vi "3_Cell_Test.vi"() -> ()   [LabVIEW 2020]
uses:
  Drivers-Essentials/global stop1.vi
  Drivers-Essentials/Global Stop 2.vi
  Global_Stop_3.vi
panel:
  out "Battery 3 Current":dbl(graph)
  out "Battery 1 Current":dbl(graph)
  out "Battery 3 Temperature":dbl(graph)
  out "Battery 3 Strain":dbl(graph)
  out "Battery 3 Voltage":dbl(graph)
  out "Battery 2 Temperature":dbl(graph)
  out "Battery 2 Strain":dbl(graph)
  out "Battery 1 Temperature":dbl(graph)
  out "Battery 1 Strain":dbl(graph)
  out "Battery 2 Voltage":dbl(graph)
  out "Battery 1 Voltage":dbl(graph)
  out "Battery 2 Current":dbl(graph)
  out "PS VIS resource name out 3":refnum<visa-resource-name>
  out "PS error out 3":errorcluster
  in  "NHR error in 3":errorcluster
  out "PS VIS resource name out 2":refnum<visa-resource-name>
  out "PS error out 2":errorcluster
  in  "NHR error in 2":errorcluster
  out "PS error out":errorcluster
  out "PS VIS resource name out":refnum<visa-resource-name>
  in  "NHR error in":errorcluster
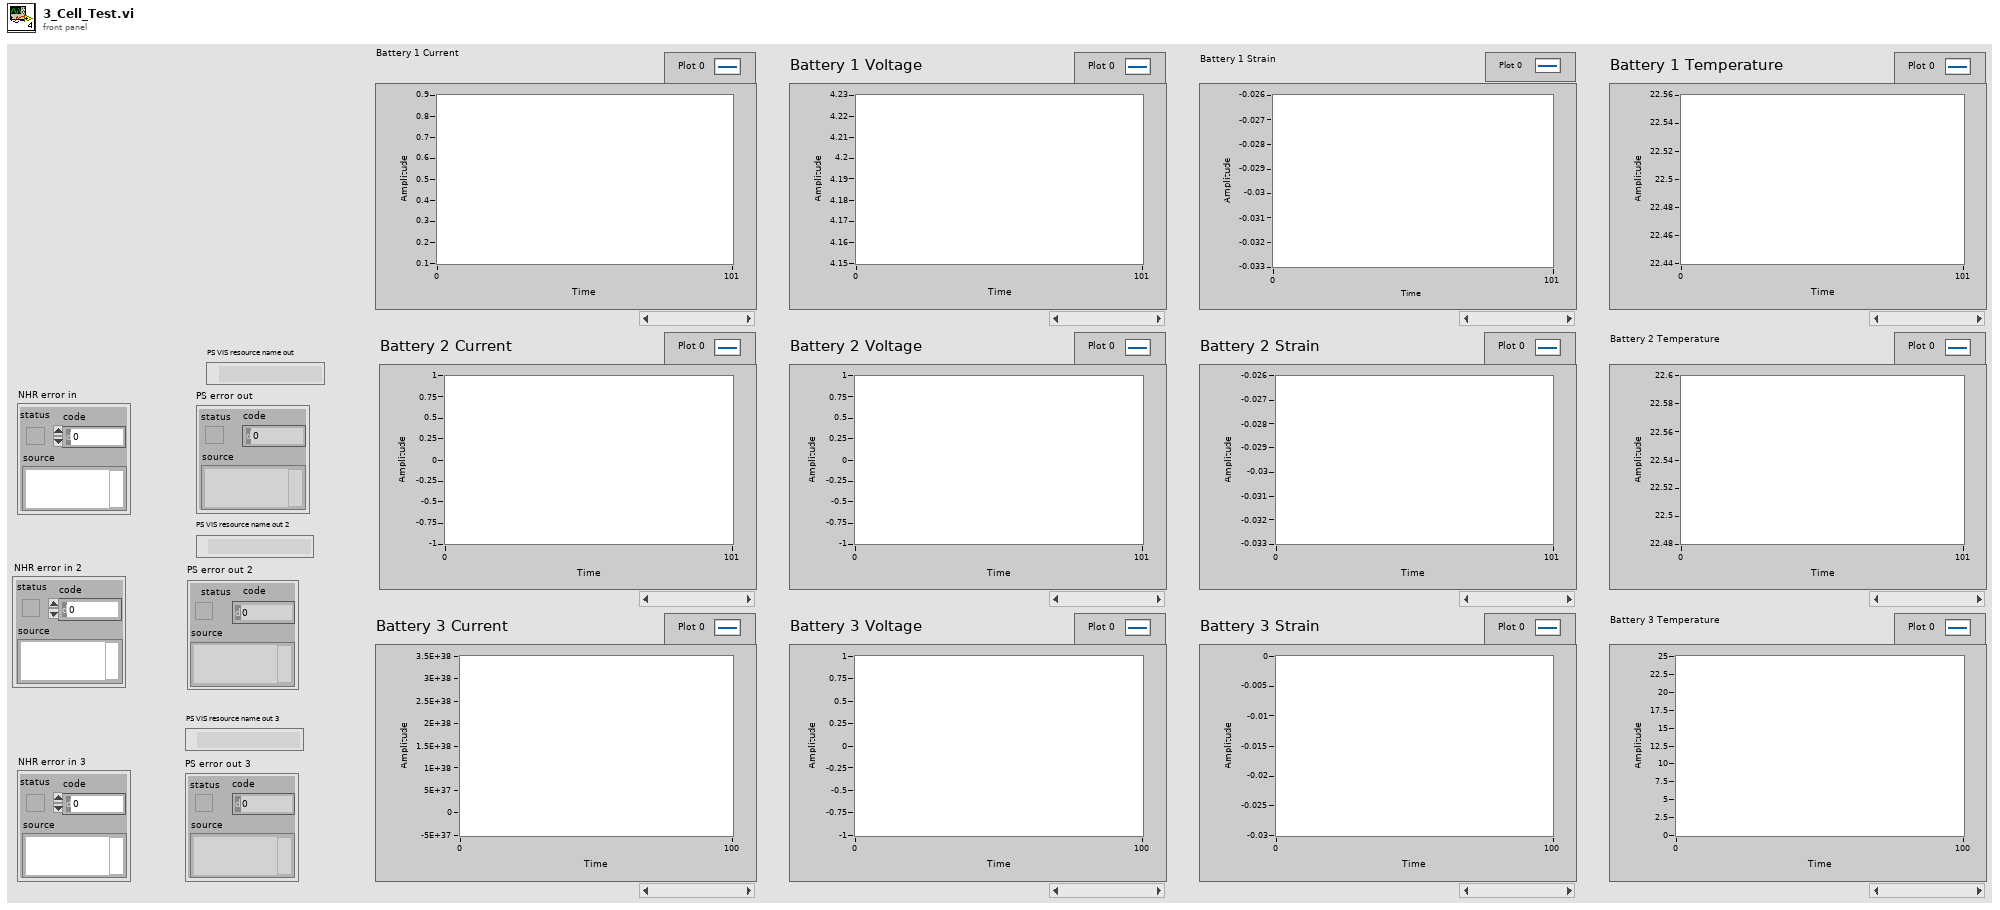
[diagram p1: front panel]
types:
  T1 = cluster{"Min Voltage (V)":dbl, "Min Voltage Time (s)":dbl, "Max Voltage (V)":dbl, "Max Voltage Time (s)":dbl, "Max Sink Current (A)":dbl, "Max Sink Current Time (s)":dbl, "Max Source Current (A)":dbl, "Max Source Current Time (s)":dbl, "Max Sink Power (W)":dbl, "Max Sink Power Time (s)":dbl, "Max Source Power (W)":dbl, "Max Source Power Time (s)":dbl}
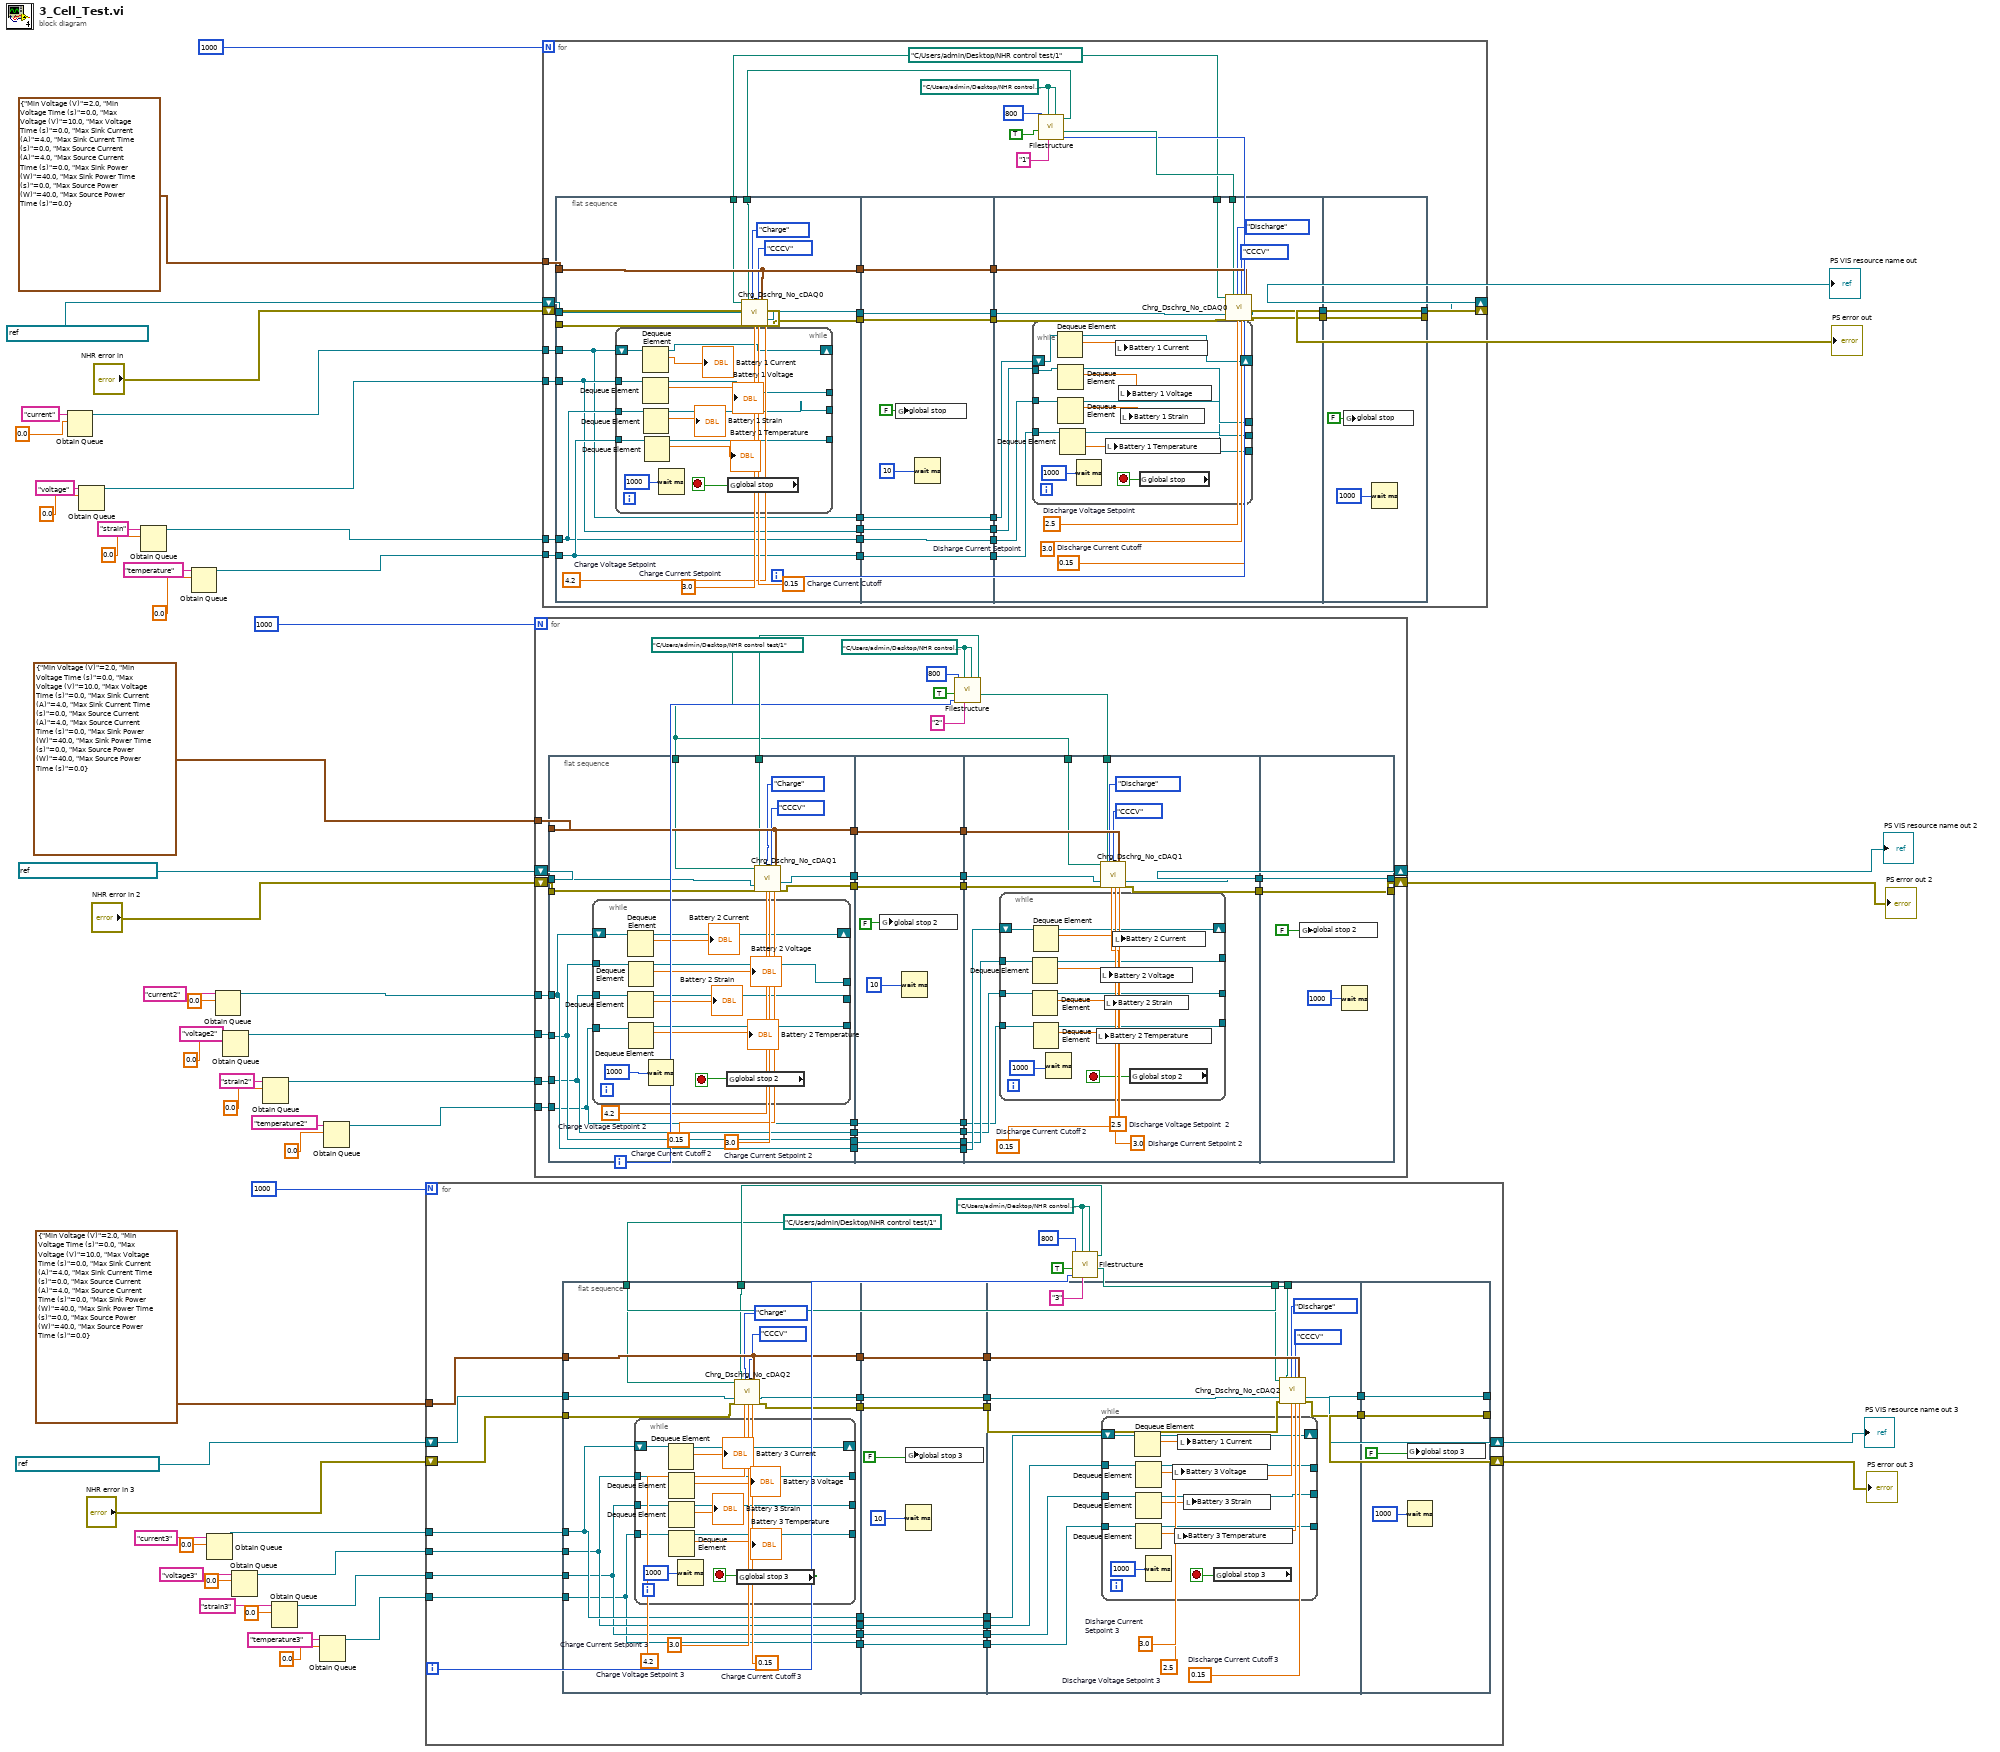
[diagram p0: block diagram]
diagram:
  n1 = Obtain Queue(name (unnamed)="current", element data type=0.0) -> (queue out=w34:refnum<queue>)  [unwired: 3 in, 2 out]
  n2 = Obtain Queue(name (unnamed)="voltage", element data type=0.0) -> (queue out=w25:refnum<queue>)  [unwired: 3 in, 2 out]
  n3 = Obtain Queue(name (unnamed)="strain", element data type=0.0) -> (queue out=w19:refnum<queue>)  [unwired: 3 in, 2 out]
  n4 = Obtain Queue(name (unnamed)="temperature", element data type=0.0) -> (queue out=w16:refnum<queue>)  [unwired: 3 in, 2 out]
  n5 = Obtain Queue(name (unnamed)="current3", element data type=0.0) -> (queue out=w28:refnum<queue>)  [unwired: 3 in, 2 out]
  n6 = Obtain Queue(name (unnamed)="current2", element data type=0.0) -> (queue out=w31:refnum<queue>)  [unwired: 3 in, 2 out]
  n7 = Obtain Queue(name (unnamed)="voltage2", element data type=0.0) -> (queue out=w22:refnum<queue>)  [unwired: 3 in, 2 out]
  n8 = Obtain Queue(name (unnamed)="voltage3", element data type=0.0) -> (queue out=w7:refnum<queue>)  [unwired: 3 in, 2 out]
  n9 = Obtain Queue(name (unnamed)="strain2", element data type=0.0) -> (queue out=w13:refnum<queue>)  [unwired: 3 in, 2 out]
  n10 = Obtain Queue(name (unnamed)="strain3", element data type=0.0) -> (queue out=w4:refnum<queue>)  [unwired: 3 in, 2 out]
  n11 = Obtain Queue(name (unnamed)="temperature3", element data type=0.0) -> (queue out=w1:refnum<queue>)  [unwired: 3 in, 2 out]
  n12 = Obtain Queue(name (unnamed)="temperature2", element data type=0.0) -> (queue out=w10:refnum<queue>)  [unwired: 3 in, 2 out]
  n13 = for {
    N: 1000 -> [_]
    tunnel: T1 {"Min Voltage (V)"=2.0, "Min Voltage Time (s)"=0.0, "Max Voltage (V)"=10.0, "Max Voltage Time (s)"=0.0, "Max Sink Current (A)"=4.0, "Max Sink Current Time (s)"=0.0, "Max Source Current (A)"=4.0, "Max Source Current Time (s)"=0.0, "Max Sink Power (W)"=40.0, "Max Sink Power Time (s)"=0.0, "Max Source Power (W)"=40.0, "Max Source Power Time (s)"=0.0} ("Output Safety") -> [w79]
    shift-right: [w85] -> w44
    shift-left: "NHR error in 3" -> [w87]
    shift-right: [w84] -> w43
    shift-left: refnum<visa-resource-name> "TCPIP0::192.168.0.94::inst0::INSTR" ("NHR VISA 3") -> [w86]
    tunnel: w28 -> [w64]
    tunnel: w7 -> [w63]
    tunnel: w4 -> [w60]
    tunnel: w1 -> [w57]
    i -> [w76]
    w75 = path "C:/Users/admin/Desktop/NHR control test/1" ("file path (use dialog)")
    w80 = path "C:/Users/admin/Desktop/NHR control test" ("filepath 3")
    n14 = flat-sequence {
      tunnel: [w103] -> w74
      tunnel: [w102] -> w72
      tunnel: [w101] -> w70
      tunnel: w79 -> [w103]
      tunnel: w87 -> [w95]
      tunnel: w86 -> [w94]
      tunnel: w78 -> [w93]
      tunnel: w75 -> [w92]
      tunnel: w64 -> [w91]
      tunnel: [w91] -> w68
      tunnel: w63 -> [w90]
      tunnel: [w90] -> w61
      tunnel: w60 -> [w89]
      tunnel: [w89] -> w58
      tunnel: w57 -> [w88]
      tunnel: [w88] -> w55
      tunnel: w74 -> [w126]
      tunnel: [w126] -> w73
      tunnel: w72 -> [w125]
      tunnel: [w125] -> w71
      tunnel: w70 -> [w124]
      tunnel: [w124] -> w69
      tunnel: w68 -> [w123]
      tunnel: [w123] -> w67
      tunnel: [w120] -> w62
      tunnel: w61 -> [w120]
      tunnel: [w119] -> w59
      tunnel: w58 -> [w119]
      tunnel: [w118] -> w56
      tunnel: w55 -> [w118]
      tunnel: w73 -> [w137]
      tunnel: w71 -> [w134]
      tunnel: w69 -> [w133]
      tunnel: w77 -> [w132]
      tunnel: w75 -> [w131]
      tunnel: w67 -> [w129]
      tunnel: [w139] -> w66
      tunnel: [w138] -> w65
      tunnel: w62 -> [w130]
      tunnel: w59 -> [w127]
      tunnel: w56 -> [w128]
      tunnel: [w159] -> w84
      tunnel: [w160] -> w85
      tunnel: w66 -> [w160]
      tunnel: w65 -> [w159]
      frame #0 {
        w100 = 0.15  # Charge Current Cutoff 3
        w99 = 3.0  # Charge Current Setpoint 3
        w98 = 4.2  # Charge Voltage Setpoint 3
        n15 = while {
          tunnel: [w115] -> _
          tunnel: [w114] -> _
          tunnel: [w113] -> _
          shift-right: [w108] -> _
          shift-left: w91 -> [w109]
          tunnel: w90 -> [w107]
          tunnel: w88 -> [w106]
          tunnel: w89 -> [w105]
          stop <- w116 stop-if-true
          n16 = Dequeue Element(queue=w109) -> (queue out=w108:refnum<queue>, element=→"Battery 3 Current":dbl)  [unwired: 2 in, 2 out]
          n17 = Dequeue Element(queue=w107) -> (queue out=w115:refnum<queue>, element=→"Battery 3 Voltage":dbl)  [unwired: 2 in, 2 out]
          n18 = Dequeue Element(queue=w105) -> (queue out=w114:refnum<queue>, element=→"Battery 3 Strain":dbl)  [unwired: 2 in, 2 out]
          n19 = Dequeue Element(queue=w106) -> (queue out=w113:refnum<queue>, element=→"Battery 3 Temperature":dbl)  [unwired: 2 in, 2 out]
          n20 = Wait (ms)(milliseconds to wait=1000) -> ()  [unwired: 1 out]
          n21 = global read "Global_Stop_3.vi" "global stop 3"() -> (w116:bool)
        }
        n22 = call "Chrg_Dschrg_No_cDAQ2.vi"("file path (use dialog)"=w92, "PS VISA in"=w94, "PS error in"=w95, "DischargeCyclePath"=w93, "Charge/discharge"=enum8{"Charge", "Discharge"}."Charge", "Charge/Discharge Voltage Setpoint"=w98, "CC or CCCV"=enum16{"CC", "CCCV"}."CCCV", "Current Setpoint"=w99, "Output Safety"=w103, "Current Cutoff"=w100) -> ("PS VIS resource name out"=w102:refnum<visa-resource-name>, "PS error out"=w101:errorcluster)  [unwired: 8 in]
      }
      frame #1 {
        n23 = global write "Global_Stop_3.vi" "global stop 3"(FALSE ("global stop")) -> ()
        n24 = Wait (ms)(milliseconds to wait=10) -> ()  [unwired: 1 out]
      }
      frame #2 {
        w141 = 3.0  # Disharge Current Setpoint 3
        w142 = 0.15  # Discharge Current Cutoff 3
        w140 = 2.5  # Discharge Voltage Setpoint 3
        n25 = while {
          tunnel: [w154] -> _
          tunnel: [w152] -> _
          tunnel: [w150] -> _
          shift-right: [w147] -> _
          shift-left: w129 -> [w148]
          tunnel: w130 -> [w146]
          tunnel: w128 -> [w145]
          tunnel: w127 -> [w144]
          stop <- w155 stop-if-true
          n26 = Dequeue Element(queue=w148) -> (queue out=w147:refnum<queue>, element=w143:dbl)  [unwired: 2 in, 2 out]
          n27 = Dequeue Element(queue=w146) -> (queue out=w154:refnum<queue>, element=w153:dbl)  [unwired: 2 in, 2 out]
          n28 = Dequeue Element(queue=w144) -> (queue out=w152:refnum<queue>, element=w151:dbl)  [unwired: 2 in, 2 out]
          n29 = Dequeue Element(queue=w145) -> (queue out=w150:refnum<queue>, element=w149:dbl)  [unwired: 2 in, 2 out]
          n30 = Wait (ms)(milliseconds to wait=1000) -> ()  [unwired: 1 out]
          n31 = local write "Battery 3 Voltage"(w153) -> ()
          n32 = local write "Battery 3 Temperature"(w149) -> ()
          n33 = local write "Battery 1 Current"(w143) -> ()
          n34 = local write "Battery 3 Strain"(w151) -> ()
          n35 = global read "Global_Stop_3.vi" "global stop 3"() -> (w155:bool)
        }
        n36 = call "Chrg_Dschrg_No_cDAQ2.vi"("file path (use dialog)"=w131, "PS VISA in"=w134, "PS error in"=w133, "DischargeCyclePath"=w132, "Charge/discharge"=enum8{"Charge", "Discharge"}."Discharge", "Charge/Discharge Voltage Setpoint"=w140, "CC or CCCV"=enum16{"CC", "CCCV"}."CCCV", "Current Setpoint"=w141, "Output Safety"=w137, "Current Cutoff"=w142) -> ("PS VIS resource name out"=w138:refnum<visa-resource-name>, "PS error out"=w139:errorcluster)  [unwired: 8 in]
      }
      frame #3 {
        n37 = global write "Global_Stop_3.vi" "global stop 3"(FALSE ("global stop")) -> ()
        n38 = Wait (ms)(milliseconds to wait=1000) -> ()  [unwired: 1 out]
      }
    }
    n39 = call "Filestructure.vi"("Discharge filepath"=w80, "Batteryname"="3" ("Batteryname 3"), "Charge filepath"=w80, "For loop i"=w76, "In for loop"=TRUE, "Starting Cycle"=800 ("Starting Cycle 3")) -> ("DischargeCyclePath"=w77:path, "ChargeCyclePath"=w78:path)  [unwired: 1 in, 3 out]
  }
  "PS error out 3" <- w44
  "PS VIS resource name out 3" <- w43
  n40 = for {
    N: 1000 -> [_]
    tunnel: T1 {"Min Voltage (V)"=2.0, "Min Voltage Time (s)"=0.0, "Max Voltage (V)"=10.0, "Max Voltage Time (s)"=0.0, "Max Sink Current (A)"=4.0, "Max Sink Current Time (s)"=0.0, "Max Source Current (A)"=4.0, "Max Source Current Time (s)"=0.0, "Max Sink Power (W)"=40.0, "Max Sink Power Time (s)"=0.0, "Max Source Power (W)"=40.0, "Max Source Power Time (s)"=0.0} ("Output Safety") -> [w185]
    shift-right: [w191] -> w48
    shift-left: "NHR error in 2" -> [w193]
    shift-right: [w190] -> w47
    shift-left: refnum<visa-resource-name> "TCPIP0::192.168.0.93::inst0::INSTR" ("NHR VISA 2") -> [w192]
    tunnel: w31 -> [w163]
    tunnel: w22 -> [w172]
    tunnel: w13 -> [w171]
    tunnel: w10 -> [w166]
    i -> [w182]
    w181 = path "C:/Users/admin/Desktop/NHR control test/1" ("file path (use dialog)")
    w186 = path "C:/Users/admin/Desktop/NHR control test" ("filepath 2")
    n41 = flat-sequence {
      tunnel: [w207] -> w180
      tunnel: [w209] -> w178
      tunnel: [w208] -> w176
      tunnel: w185 -> [w209]
      tunnel: w193 -> [w202]
      tunnel: w192 -> [w203]
      tunnel: w183 -> [w199]
      tunnel: w181 -> [w198]
      tunnel: w172 -> [w196]
      tunnel: w171 -> [w195]
      tunnel: [w196] -> w169
      tunnel: [w195] -> w167
      tunnel: w166 -> [w194]
      tunnel: [w194] -> w164
      tunnel: w163 -> [w197]
      tunnel: [w197] -> w161
      tunnel: w180 -> [w232]
      tunnel: [w232] -> w179
      tunnel: w178 -> [w231]
      tunnel: [w231] -> w177
      tunnel: w176 -> [w230]
      tunnel: [w230] -> w175
      tunnel: [w227] -> w170
      tunnel: w169 -> [w227]
      tunnel: [w226] -> w168
      tunnel: w167 -> [w226]
      tunnel: [w225] -> w165
      tunnel: w164 -> [w225]
      tunnel: [w224] -> w162
      tunnel: w161 -> [w224]
      tunnel: w179 -> [w243]
      tunnel: w177 -> [w241]
      tunnel: w184 -> [w238]
      tunnel: w175 -> [w242]
      tunnel: w181 -> [w237]
      tunnel: [w245] -> w174
      tunnel: [w244] -> w173
      tunnel: w170 -> [w235]
      tunnel: w168 -> [w234]
      tunnel: w165 -> [w233]
      tunnel: w162 -> [w236]
      tunnel: [w265] -> w190
      tunnel: [w266] -> w191
      tunnel: w174 -> [w266]
      tunnel: w173 -> [w265]
      frame #0 {
        w204 = 0.15  # Charge Current Cutoff 2
        w205 = 3.0  # Charge Current Setpoint 2
        w206 = 4.2  # Charge Voltage Setpoint 2
        n42 = while {
          tunnel: [w220] -> _
          tunnel: [w218] -> _
          tunnel: [w216] -> _
          shift-right: [w213] -> _
          shift-left: w197 -> [w214]
          tunnel: w196 -> [w212]
          tunnel: w195 -> [w211]
          tunnel: w194 -> [w210]
          stop <- w221 stop-if-true
          n43 = Dequeue Element(queue=w214) -> (queue out=w213:refnum<queue>, element=→"Battery 2 Current":dbl)  [unwired: 2 in, 2 out]
          n44 = Dequeue Element(queue=w211) -> (queue out=w218:refnum<queue>, element=→"Battery 2 Strain":dbl)  [unwired: 2 in, 2 out]
          n45 = Dequeue Element(queue=w212) -> (queue out=w220:refnum<queue>, element=→"Battery 2 Voltage":dbl)  [unwired: 2 in, 2 out]
          n46 = Dequeue Element(queue=w210) -> (queue out=w216:refnum<queue>, element=→"Battery 2 Temperature":dbl)  [unwired: 2 in, 2 out]
          n47 = Wait (ms)(milliseconds to wait=1000) -> ()  [unwired: 1 out]
          n48 = global read "Global Stop 2.vi" "global stop 2"() -> (w221:bool)
        }
        n49 = call "Chrg_Dschrg_No_cDAQ1.vi"("file path (use dialog)"=w198, "PS VISA in"=w203, "PS error in"=w202, "DischargeCyclePath"=w199, "Charge/discharge"=enum8{"Charge", "Discharge"}."Charge", "Charge/Discharge Voltage Setpoint"=w206, "CC or CCCV"=enum16{"CC", "CCCV"}."CCCV", "Current Setpoint"=w205, "Output Safety"=w209, "Current Cutoff"=w204) -> ("PS VIS resource name out"=w208:refnum<visa-resource-name>, "PS error out"=w207:errorcluster)  [unwired: 8 in]
      }
      frame #1 {
        n50 = global write "Global Stop 2.vi" "global stop 2"(FALSE ("global stop")) -> ()
        n51 = Wait (ms)(milliseconds to wait=10) -> ()  [unwired: 1 out]
      }
      frame #2 {
        w247 = 3.0  # Disharge Current Setpoint 2
        w248 = 0.15  # Discharge Current Cutoff 2
        w246 = 2.5  # Discharge Voltage Setpoint  2
        n52 = while {
          tunnel: [w258] -> _
          tunnel: [w257] -> _
          tunnel: [w255] -> _
          shift-right: [w251] -> _
          shift-left: w236 -> [w252]
          tunnel: w235 -> [w253]
          tunnel: w234 -> [w250]
          tunnel: w233 -> [w249]
          stop <- w260 stop-if-true
          n53 = Dequeue Element(queue=w253) -> (queue out=w258:refnum<queue>, element=w259:dbl)  [unwired: 2 in, 2 out]
          n54 = Dequeue Element(queue=w250) -> (queue out=w257:refnum<queue>, element=w256:dbl)  [unwired: 2 in, 2 out]
          n55 = Dequeue Element(queue=w252) -> (queue out=w251:refnum<queue>, element=w261:dbl)  [unwired: 2 in, 2 out]
          n56 = Dequeue Element(queue=w249) -> (queue out=w255:refnum<queue>, element=w254:dbl)  [unwired: 2 in, 2 out]
          n57 = Wait (ms)(milliseconds to wait=1000) -> ()  [unwired: 1 out]
          n58 = local write "Battery 2 Temperature"(w254) -> ()
          n59 = local write "Battery 2 Voltage"(w259) -> ()
          n60 = local write "Battery 2 Strain"(w256) -> ()
          n61 = local write "Battery 2 Current"(w261) -> ()
          n62 = global read "Global Stop 2.vi" "global stop 2"() -> (w260:bool)
        }
        n63 = call "Chrg_Dschrg_No_cDAQ1.vi"("file path (use dialog)"=w237, "PS VISA in"=w242, "PS error in"=w243, "DischargeCyclePath"=w238, "Charge/discharge"=enum8{"Charge", "Discharge"}."Discharge", "Charge/Discharge Voltage Setpoint"=w246, "CC or CCCV"=enum16{"CC", "CCCV"}."CCCV", "Current Setpoint"=w247, "Output Safety"=w241, "Current Cutoff"=w248) -> ("PS VIS resource name out"=w244:refnum<visa-resource-name>, "PS error out"=w245:errorcluster)  [unwired: 8 in]
      }
      frame #3 {
        n64 = global write "Global Stop 2.vi" "global stop 2"(FALSE ("global stop")) -> ()
        n65 = Wait (ms)(milliseconds to wait=1000) -> ()  [unwired: 1 out]
      }
    }
    n66 = call "Filestructure.vi"("Discharge filepath"=w186, "Batteryname"="2" ("Batteryname 2"), "Charge filepath"=w186, "For loop i"=w182, "In for loop"=TRUE, "Starting Cycle"=800 ("Starting Cycle 2")) -> ("DischargeCyclePath"=w184:path, "ChargeCyclePath"=w183:path)  [unwired: 1 in, 3 out]
  }
  "PS error out 2" <- w48
  "PS VIS resource name out 2" <- w47
  n67 = for {
    N: 1000 -> [_]
    tunnel: T1 {"Min Voltage (V)"=2.0, "Min Voltage Time (s)"=0.0, "Max Voltage (V)"=10.0, "Max Voltage Time (s)"=0.0, "Max Sink Current (A)"=4.0, "Max Sink Current Time (s)"=0.0, "Max Source Current (A)"=4.0, "Max Source Current Time (s)"=0.0, "Max Sink Power (W)"=40.0, "Max Sink Power Time (s)"=0.0, "Max Source Power (W)"=40.0, "Max Source Power Time (s)"=0.0} ("Output Safety") -> [w292]
    shift-right: [w298] -> w53
    shift-left: "NHR error in" -> [w299]
    shift-right: [w297] -> w52
    shift-left: refnum<visa-resource-name> "TCPIP0::192.168.0.92::inst0::INSTR" ("NHR VISA") -> [w291]
    tunnel: w34 -> [w286]
    tunnel: w25 -> [w277]
    tunnel: w19 -> [w276]
    tunnel: w16 -> [w275]
    i -> [w288]
    w287 = path "C:/Users/admin/Desktop/NHR control test/1" ("file path (use dialog)")
    w293 = path "C:/Users/admin/Desktop/NHR control test" ("filepath")
    n68 = flat-sequence {
      tunnel: [w314] -> w285
      tunnel: [w315] -> w283
      tunnel: [w313] -> w281
      tunnel: w292 -> [w313]
      tunnel: w299 -> [w309]
      tunnel: w291 -> [w308]
      tunnel: w289 -> [w305]
      tunnel: w287 -> [w304]
      tunnel: w286 -> [w300]
      tunnel: w277 -> [w301]
      tunnel: w276 -> [w302]
      tunnel: w275 -> [w303]
      tunnel: [w303] -> w273
      tunnel: [w302] -> w271
      tunnel: [w301] -> w269
      tunnel: [w300] -> w267
      tunnel: w285 -> [w338]
      tunnel: [w338] -> w284
      tunnel: w283 -> [w337]
      tunnel: [w337] -> w282
      tunnel: w281 -> [w336]
      tunnel: [w336] -> w280
      tunnel: [w333] -> w274
      tunnel: w273 -> [w333]
      tunnel: [w332] -> w272
      tunnel: w271 -> [w332]
      tunnel: [w331] -> w270
      tunnel: w269 -> [w331]
      tunnel: [w330] -> w268
      tunnel: w267 -> [w330]
      tunnel: w284 -> [w349]
      tunnel: w282 -> [w348]
      tunnel: w290 -> [w346]
      tunnel: w280 -> [w347]
      tunnel: w287 -> [w343]
      tunnel: [w351] -> w279
      tunnel: [w350] -> w278
      tunnel: w274 -> [w341]
      tunnel: w272 -> [w342]
      tunnel: w270 -> [w340]
      tunnel: w268 -> [w339]
      tunnel: [w371] -> w297
      tunnel: [w372] -> w298
      tunnel: w279 -> [w372]
      tunnel: w278 -> [w371]
      frame #0 {
        w312 = 0.15  # Charge Current Cutoff
        w311 = 3.0  # Charge Current Setpoint
        w310 = 4.2  # Charge Voltage Setpoint
        n69 = while {
          tunnel: [w327] -> _
          tunnel: [w325] -> _
          tunnel: [w323] -> _
          shift-right: [w317] -> _
          shift-left: w300 -> [w321]
          tunnel: w301 -> [w320]
          tunnel: w303 -> [w319]
          tunnel: w302 -> [w318]
          stop <- w328 stop-if-true
          n70 = Dequeue Element(queue=w321) -> (queue out=w317:refnum<queue>, element=→"Battery 1 Current":dbl)  [unwired: 2 in, 2 out]
          n71 = Dequeue Element(queue=w320) -> (queue out=w327:refnum<queue>, element=→"Battery 1 Voltage":dbl)  [unwired: 2 in, 2 out]
          n72 = Dequeue Element(queue=w318) -> (queue out=w325:refnum<queue>, element=→"Battery 1 Strain":dbl)  [unwired: 2 in, 2 out]
          n73 = Dequeue Element(queue=w319) -> (queue out=w323:refnum<queue>, element=→"Battery 1 Temperature":dbl)  [unwired: 2 in, 2 out]
          n74 = Wait (ms)(milliseconds to wait=1000) -> ()  [unwired: 1 out]
          n75 = global read "global stop1.vi" "global stop"() -> (w328:bool)
        }
        n76 = call "Chrg_Dschrg_No_cDAQ0.vi"("file path (use dialog)"=w304, "PS VISA in"=w308, "PS error in"=w309, "DischargeCyclePath"=w305, "Charge/discharge"=enum8{"Charge", "Discharge"}."Charge", "Charge/Discharge Voltage Setpoint"=w310, "CC or CCCV"=enum16{"CC", "CCCV"}."CCCV", "Current Setpoint"=w311, "Output Safety"=w313, "Current Cutoff"=w312) -> ("PS VIS resource name out"=w315:refnum<visa-resource-name>, "PS error out"=w314:errorcluster)  [unwired: 8 in]
      }
      frame #1 {
        n77 = global write "global stop1.vi" "global stop"(FALSE ("global stop")) -> ()
        n78 = Wait (ms)(milliseconds to wait=10) -> ()  [unwired: 1 out]
      }
      frame #2 {
        w353 = 3.0  # Disharge Current Setpoint
        w354 = 0.15  # Discharge Current Cutoff
        w352 = 2.5  # Discharge Voltage Setpoint
        n79 = while {
          tunnel: [w366] -> _
          tunnel: [w364] -> _
          tunnel: [w362] -> _
          shift-right: [w356] -> _
          shift-left: w339 -> [w357]
          tunnel: w342 -> [w360]
          tunnel: w341 -> [w359]
          tunnel: w340 -> [w358]
          stop <- w367 stop-if-true
          n80 = Dequeue Element(queue=w357) -> (queue out=w356:refnum<queue>, element=w355:dbl)  [unwired: 2 in, 2 out]
          n81 = Dequeue Element(queue=w358) -> (queue out=w366:refnum<queue>, element=w365:dbl)  [unwired: 2 in, 2 out]
          n82 = Dequeue Element(queue=w360) -> (queue out=w364:refnum<queue>, element=w363:dbl)  [unwired: 2 in, 2 out]
          n83 = Dequeue Element(queue=w359) -> (queue out=w362:refnum<queue>, element=w361:dbl)  [unwired: 2 in, 2 out]
          n84 = Wait (ms)(milliseconds to wait=1000) -> ()  [unwired: 1 out]
          n85 = local write "Battery 1 Temperature"(w361) -> ()
          n86 = local write "Battery 1 Current"(w355) -> ()
          n87 = local write "Battery 1 Voltage"(w365) -> ()
          n88 = local write "Battery 1 Strain"(w363) -> ()
          n89 = global read "global stop1.vi" "global stop"() -> (w367:bool)
        }
        n90 = call "Chrg_Dschrg_No_cDAQ0.vi"("file path (use dialog)"=w343, "PS VISA in"=w348, "PS error in"=w349, "DischargeCyclePath"=w346, "Charge/discharge"=enum8{"Charge", "Discharge"}."Discharge", "Charge/Discharge Voltage Setpoint"=w352, "CC or CCCV"=enum16{"CC", "CCCV"}."CCCV", "Current Setpoint"=w353, "Output Safety"=w347, "Current Cutoff"=w354) -> ("PS VIS resource name out"=w350:refnum<visa-resource-name>, "PS error out"=w351:errorcluster)  [unwired: 8 in]
      }
      frame #3 {
        n91 = global write "global stop1.vi" "global stop"(FALSE ("global stop")) -> ()
        n92 = Wait (ms)(milliseconds to wait=1000) -> ()  [unwired: 1 out]
      }
    }
    n93 = call "Filestructure.vi"("Discharge filepath"=w293, "Batteryname"="1", "Charge filepath"=w293, "For loop i"=w288, "In for loop"=TRUE, "Starting Cycle"=800) -> ("DischargeCyclePath"=w290:path, "ChargeCyclePath"=w289:path)  [unwired: 1 in, 3 out]
  }
  "PS error out" <- w53
  "PS VIS resource name out" <- w52
